vi "Create Attribute Section and Channels.vi"(8 "error in (no error)":errorcluster, 9 "Type":T1, 10 "Item Ref":T4 format="%.0x", 11 "Channel Configuration":T2) -> (0 "error out":errorcluster)   [LabVIEW 2023, in "Ethernet IP Custom Device Custom Device.lvlib"]
uses:
  Ethernet IP Custom Device Custom Device.lvlib
  <vilib>/NI VeriStand/Custom Device API/Custom Device Item Ref.ctl
  EIP Attribute Channel Info.ctl
  EIP Attribute Direction.ctl
  <vilib>/NI VeriStand/Custom Device API/Custom Device Channel Type.ctl
  EIP Message Type.ctl
  <vilib>/NI VeriStand/Custom Device API/Custom Device Channel.ctl
  Ethernet IP Global Strings.vi
  <vilib>/NI VeriStand/Custom Device API/Set Item Property (U32).vi
  Ethernet IP Global GUIDs.vi
  <vilib>/NI VeriStand/Custom Device API/Custom Device API.lvlib
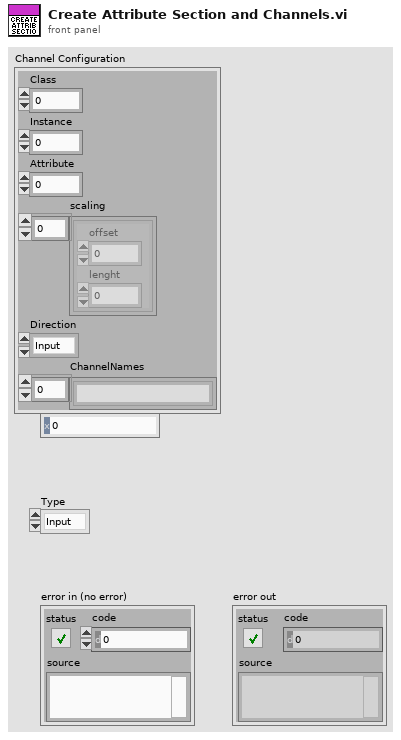
[diagram p1: front panel]
types:
  T1 = typedef "Custom Device API.lvlib/Custom Device Channel Type.ctl" = enum16{"Input", "Output"}
  T2 = typedef "Ethernet IP Custom Device Custom Device.lvlib/EIP Attribute Channel Info.ctl" = cluster{"Class":i32, "Instance":u32, "Attribute":i32, "scaling":cluster{"offset":u32, "lenght":u32}[], "Direction":T3, "ChannelNames":string[]}
  T3 = typedef "Ethernet IP Custom Device Custom Device.lvlib/EIP Attribute Direction.ctl" = enum16{"Input", "Output"}
  T4 = typedef "Custom Device API.lvlib/Custom Device Item Ref.ctl" = u64
  T5 = typedef "Ethernet IP Custom Device Custom Device.lvlib/EIP Message Type.ctl" = enum16{"Tag", "Assembly"}
  T6 = typedef "Custom Device API.lvlib/Custom Device Channel.ctl" = cluster{"Type":T1, "Units":string, "Default Value":dbl, "Faultable":bool, "Scalable":bool}
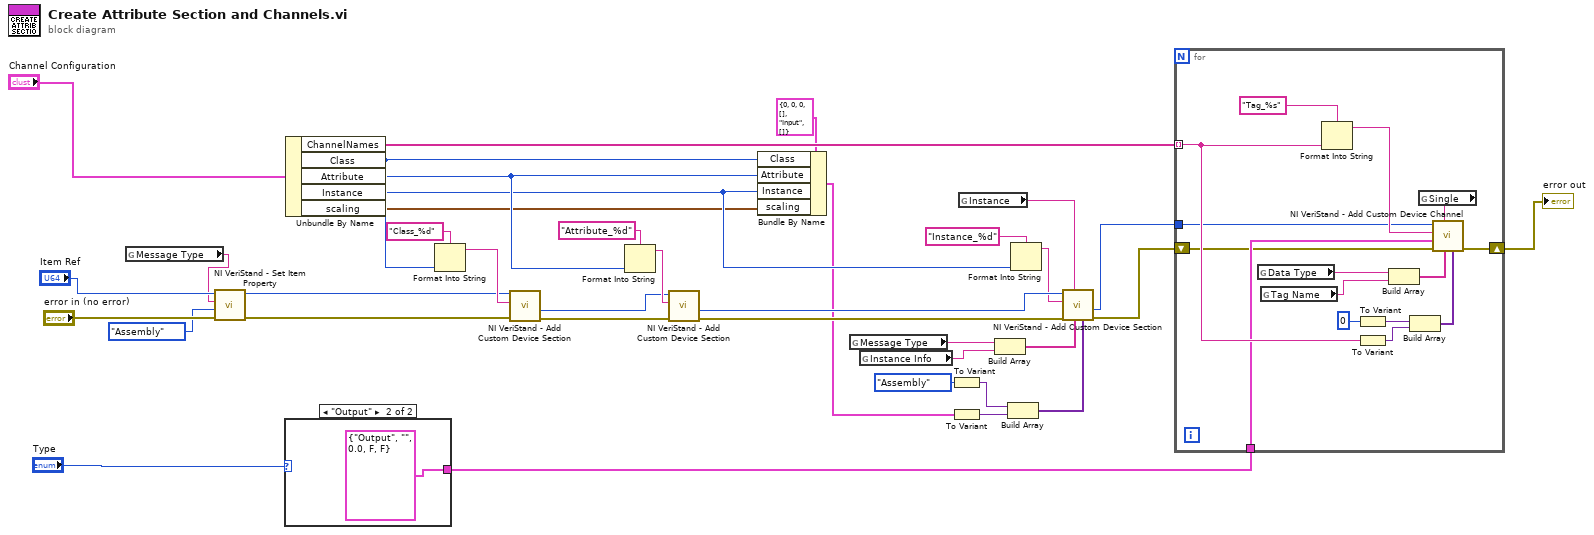
[diagram p0: block diagram]
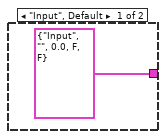
[diagram p2: hidden frame]
diagram:
  n1 = global read "Ethernet IP Global Strings.vi" "Message Type"() -> (w3:string)
  n2 = call-poly <vilib>:"NI VeriStand - Set Item Property.vi"("error in (no error)"="error in (no error)", "Value"=EIP_Message_Type."Assembly" ("Message Type"), "Property Name"=w3, "Item Ref in"="Item Ref") -> ("error out"=w5:errorcluster, "Item Ref out"=w4:T4)  [unwired: 5 in, 1 out]
  n3 = case shown="\"Output\"" "Type" {
    tunnel: [T6 {"Type"=enum."Input", "Units"="", "Default Value"=0.0, "Faultable"=FALSE, "Scalable"=FALSE} ("Channel") T6 {"Type"=enum."Output", "Units"="", "Default Value"=0.0, "Faultable"=FALSE, "Scalable"=FALSE} ("Channel")] -> w32
    frame "Input", Default {
    }
    frame "Output" {
    }
  }
  n4 = Unbundle By Name("Channel Configuration") -> ("ChannelNames"=w37:string[], "Class"=w30:i32, "Attribute"=w26:i32, "Instance"=w25:u32, "scaling"=w10:cluster{"offset":u32, "lenght":u32}[])
  n5 = Format Into String(format string="Class_%d", w30) -> (resulting string=w29:string)  [unwired: 2 in, 1 out]
  n6 = call <vilib>:"NI VeriStand - Add Custom Device Section.vi"("error in (no error)"=w5, "Section Name"=w29, "Parent Ref in"=w4) -> ("error out"=w20:errorcluster, "Section Ptr"=w23:T4)  [unwired: 5 in, 2 out]
  n7 = Format Into String(format string="Attribute_%d", w26) -> (resulting string=w24:string)  [unwired: 2 in, 1 out]
  n8 = call <vilib>:"NI VeriStand - Add Custom Device Section.vi"("error in (no error)"=w20, "Section Name"=w24, "Parent Ref in"=w23) -> ("error out"=w19:errorcluster, "Section Ptr"=w22:T4)  [unwired: 5 in, 2 out]
  n9 = Bundle By Name(cluster=T2 {"Class"=0, "Instance"=0, "Attribute"=0, "scaling"=[], "Direction"=enum."Input", "ChannelNames"=[]} ("Attribute Info"), "Class"=w30, "Attribute"=w26, "Instance"=w25, "scaling"=w10) -> (w9:T2)
  n10 = global read "Ethernet IP Global Strings.vi" "Message Type"() -> (w18:string)
  n11 = global read "Ethernet IP Global Strings.vi" "Instance Info"() -> (w17:string)
  n12 = To Variant(anything=EIP_Message_Type."Assembly" ("Message Type")) -> (Variant=w15:variant)
  n13 = To Variant(anything=w9) -> (Variant=w14:variant)
  n14 = global read "Ethernet IP Global GUIDs.vi" "Instance"() -> (w1:string)
  n15 = Build Array(w18, w17) -> (w16:string[])
  n16 = Build Array(w15, w14) -> (w8:variant[])
  n17 = Format Into String(format string="Instance_%d", w25) -> (resulting string=w21:string)  [unwired: 2 in, 1 out]
  n18 = call <vilib>:"NI VeriStand - Add Custom Device Section.vi"("Property Values"=w8, "Property names"=w16, "GUID (Default Section)"=w1, "error in (no error)"=w19, "Section Name"=w21, "Parent Ref in"=w22) -> ("error out"=w11:errorcluster, "Section Ptr"=w12:T4)  [unwired: 2 in, 2 out]
  n19 = for {
    tunnel: w37 -> [w54] mode=indexing
    tunnel: w32 -> [w45]
    tunnel: w12 -> [w41]
    shift-right: [w47] -> w35
    shift-left: w11 -> [w40]
    n20 = global read "Ethernet IP Global Strings.vi" "Data Type"() -> (w48:string)
    n21 = global read "Ethernet IP Global Strings.vi" "Tag Name"() -> (w49:string)
    n22 = Format Into String(format string="Tag_%s", w54) -> (resulting string=w53:string)  [unwired: 2 in, 1 out]
    n23 = To Variant(anything=u16 0) -> (Variant=w42:variant)
    n24 = To Variant(anything=w54) -> (Variant=w43:variant)
    n25 = Build Array(w48, w49) -> (w44:string[])
    n26 = Build Array(w42, w43) -> (w50:variant[])
    n27 = global read "Ethernet IP Global GUIDs.vi" "Single"() -> (w46:string)
    n28 = call <vilib>:"NI VeriStand - Add Custom Device Channel.vi"("Property Values"=w50, "Property names"=w44, "GUID (Default Channel)"=w46, "error in (no error)"=w40, "Channel"=w45, "Channel Name"=w53, "Parent Ref in"=w41) -> ("error out"=w47:errorcluster)  [unwired: 1 in, 3 out]
  }
  "error out" <- w35
